vi "add_steering_is.vi"(1 "steering_is":T1, 2 "msg in":string) -> (0 "msg out":string)   [LabVIEW 2016]
uses:
  <userlib>/ROS for LabVIEW Software/ROS/MessageBuilding/std_msgs/subs/float64Scalar.vi
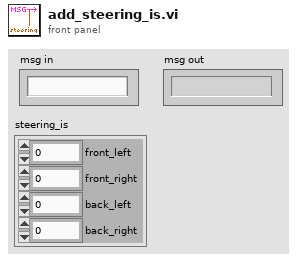
[diagram p1: front panel]
types:
  T1 = cluster{"front_left":dbl, "front_right":dbl, "back_left":dbl, "back_right":dbl}
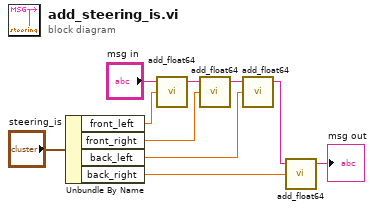
[diagram p0: block diagram]
diagram:
  n1 = Unbundle By Name("steering_is") -> ("front_left"=w4:dbl, "front_right"=w3:dbl, "back_left"=w2:dbl, "back_right"=w1:dbl)
  n2 = call-poly <userlib>:"add_float64.vi"("Numeric"=w4, "msg in"="msg in") -> ("msg out"=w8:string)  [unwired: 3 in]
  n3 = call-poly <userlib>:"add_float64.vi"("Numeric"=w3, "msg in"=w8) -> ("msg out"=w7:string)  [unwired: 3 in]
  n4 = call-poly <userlib>:"add_float64.vi"("Numeric"=w2, "msg in"=w7) -> ("msg out"=w6:string)  [unwired: 3 in]
  n5 = call-poly <userlib>:"add_float64.vi"("Numeric"=w1, "msg in"=w6) -> ("msg out"=→"msg out":string)  [unwired: 3 in]
